vi "NeedleValveOpen.vi"(8 "error in (no error)":errorcluster, 10 "Percent Difference":i32, 11 "VISA resource name":refnum<visa-resource-name>) -> (0 "error out":errorcluster, 3 "VISA resource name out":refnum<visa-resource-name>)   [LabVIEW 2017]
uses:
  <instrlib>/zabertseries/Public/Utility/Request.ctl
  <instrlib>/zabertseries/ZaberTSeries.lvlib
panel:
  out "data":dbl
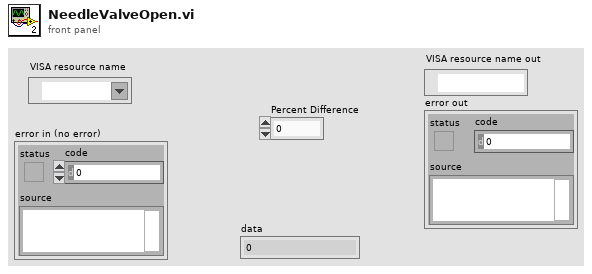
[diagram p1: front panel]
types:
  T1 = typedef "ZaberTSeries.lvlib/Request.ctl" = cluster{"Device Number":u8, "Command":u8, "Data":i32, "Response Count":i32}
  T2 = cluster{"Device Number":u8, "Command":u8, i32, "Response Count":i32}
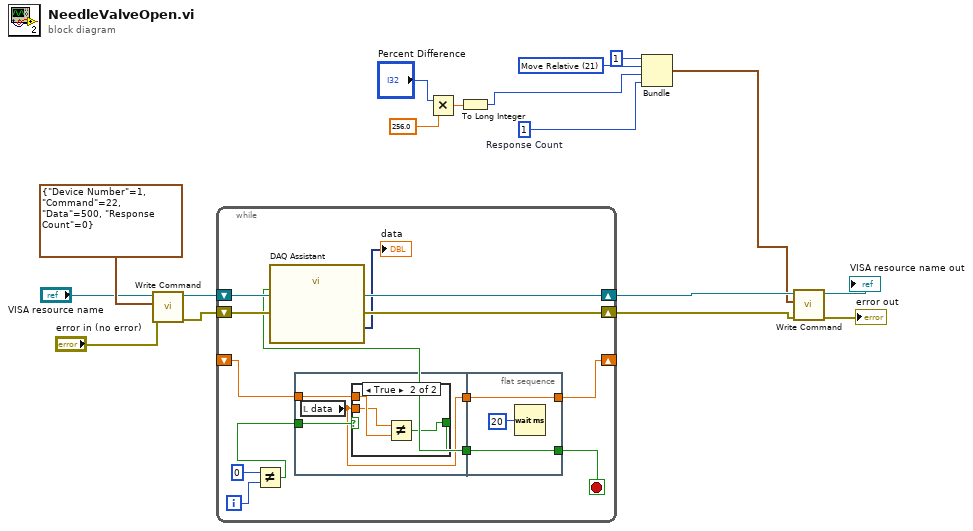
[diagram p0: block diagram]
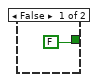
[diagram p2: hidden frame]
diagram:
  w7 = 1  # Response Count
  w8 = u8 21 items=["Echo"=55, "Home"=1, "Move Absolute"=20, "Move Relative"=21, "Move at Constant Speed"=22, "Renumber"=2, "Restore Settings"=36, "Stop"=23] ("Command")
  n1 = call <instrlib>:"Write Command.vi"("error in (no error)"="error in (no error)", "Request"=T1 {"Device Number"=1, "Command"=22, "Data"=500, "Response Count"=0}, "VISA resource name"="VISA resource name") -> ("error out"=w14:errorcluster, "VISA resource name out"=w15:refnum<visa-resource-name>)  [unwired: 6 in, 1 out]
  n2 = while {
    shift-right: [w28] -> w13
    shift-left: w15 -> [w28]
    shift-right: [w27] -> w12
    shift-left: w14 -> [w27]
    shift-right: [w18] -> _
    shift-left: _ -> [w25]
    i -> [w23]
    stop <- w26 stop-if-true
    n3 = Not Equal?(x=0, y=w23) -> (x != y?=w21:bool)
    n4 = call "DAQ Assistant"("stop (F)"=w26) -> ("data"=→"data":dynamicdata)  [unwired: 15 in, 3 out]
    n5 = flat-sequence {
      tunnel: w25 -> [w31]
      tunnel: w21 -> [w30]
      tunnel: [w32] -> w20
      tunnel: [w29] -> w19
      tunnel: [w39] -> w26
      tunnel: w20 -> [w39]
      tunnel: [w37] -> w18
      tunnel: w19 -> [w37]
      frame #0 {
        n6 = local read "data"() -> (w29:dbl)
        n7 = case shown="True" w30 {
          tunnel: [FALSE w36] -> w32
          tunnel: w31 -> [_ w35]
          tunnel: w29 -> [_ w34]
          frame False {
          }
          frame True {
            n8 = Not Equal?(x=w34, y=w35) -> (x != y?=w36:bool)
          }
        }
      }
      frame #1 {
        n9 = Wait (ms)(milliseconds to wait=u32 20) -> ()  [unwired: 1 out]
      }
    }
  }
  n10 = Multiply(x="Percent Difference", y=256.0) -> (x*y=w4:dbl)
  n11 = To Long Integer(number=w4) -> (32bit integer=w3:i32)
  n12 = Bundle("Device Number"=u8 1, "Command"=w8, w3, "Response Count"=w7) -> (w1:T2)  [unwired: 1 in]
  n13 = call <instrlib>:"Write Command.vi"("error in (no error)"=w12, "Request"=w1, "VISA resource name"=w13) -> ("error out"=→"error out":errorcluster, "VISA resource name out"=→"VISA resource name out":refnum<visa-resource-name>)  [unwired: 6 in, 1 out]
